vi "Set Wait time.vi"(8 "error in (no error)":errorcluster, 11 "ia test param in":refnum<class "IA Test Parameters.lvclass">) -> (0 "error out":errorcluster, 3 "ia test param out":refnum<class "IA Test Parameters.lvclass">)   [LabVIEW 2020]
uses:
  Parameter Class/IA Test Parameters.lvclass
  Parameter Class/IA Test Parameters.lvclass/IA Test Parameters.ctl
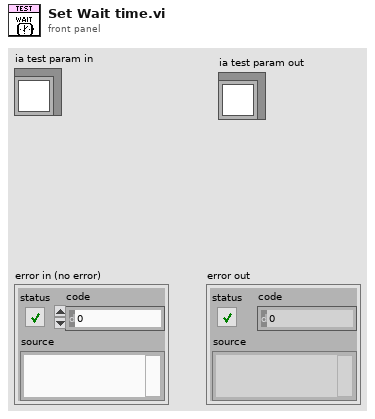
[diagram p1: front panel]
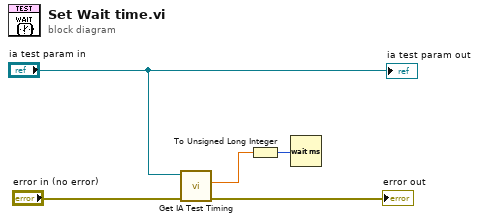
[diagram p0: block diagram]
diagram:
  n1 = call "Get IA Test Timing.vi"("error in (no error)"="error in (no error)", "IA Test Parameters in"="ia test param in") -> ("error out"=→"error out":errorcluster, "loop wait (ms)"=w2:dbl)  [unwired: 4 in, 4 out]
  n2 = To Unsigned Long Integer(number=w2) -> (unsigned 32bit integer=w3:u32)
  n3 = Wait (ms)(milliseconds to wait=w3) -> ()  [unwired: 1 out]
  "ia test param out" <- "ia test param in"
